vi "Cleanup.vi"(8 "error in (no error)":errorcluster, 11 "Vecto in":refnum<class "Vecto.lvclass">) -> (0 "error out":errorcluster)   [LabVIEW 2020, in "Vecto.lvlib" / "Vecto.lvclass"]
uses:
  Vecto.lvclass
  lv-http-server/HTTP Server/Server/Server.lvclass
  VectoService/VectoInfo.lvclass
  InfoService/NodeStatus.lvclass
  DiscoveryService/DiscoveryService.lvclass
  SequenceCountService/SequenceCountService.lvclass
  RemoteDataService/RemoteDataService.lvclass
  ChannelService/ChannelService.lvclass
  TCPMessaging/TCPMessaging.lvclass
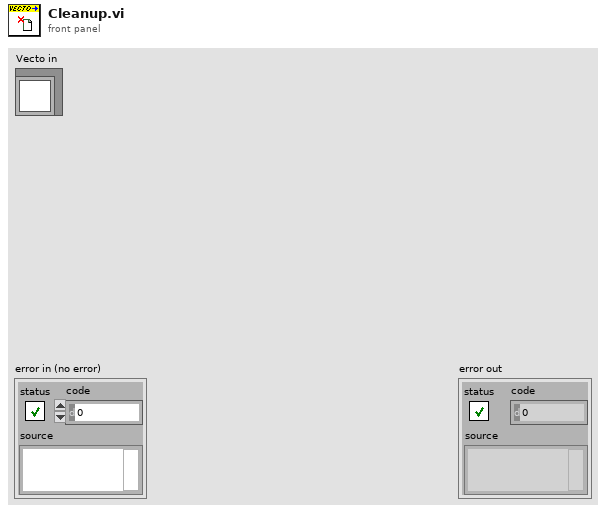
[diagram p1: front panel]
types:
  T1 = typedef "Vecto.lvlib/Vecto.lvclass/Local Services.ctl" = cluster{"InfoService":refnum<class "NodeStatus.lvclass">, "VectoService":refnum<class "VectoInfo.lvclass">, "ChannelService":refnum<class "ChannelService.lvclass">, "EventLogging":refnum<class "EventLoggingService.lvclass">}
  T2 = typedef "Vecto.lvlib/Vecto.lvclass/Remote Services.ctl" = cluster{"DiscoveryService":refnum<class "DiscoveryService.lvclass">, "SequenceCountService":refnum<class "SequenceCountService.lvclass">, "RemoteDataService":refnum<class "RemoteDataService.lvclass">, "TCPMessaging":refnum<class "TCPMessaging.lvclass">}
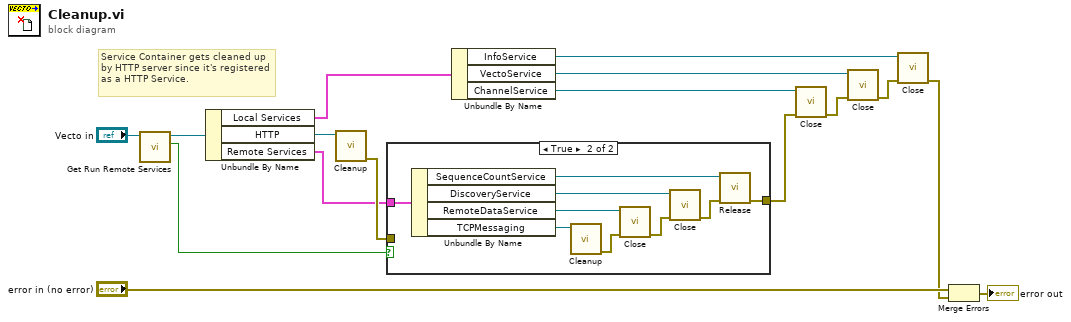
[diagram p0: block diagram]
diagram:
  # "Service Container gets cleaned up by HTTP server since it's registered as a HTTP Service."
  n1 = call "Get Run Remote Services.vi"("Vecto in"="Vecto in") -> ("Run Remote Services"=w7:bool, "Vecto out"=w8:refnum<class "Vecto.lvclass">)  [unwired: 8 in, 1 out]
  n2 = Unbundle By Name(w8) -> ("Local Services"=w14:T1, "HTTP"=w15:refnum<class "Server.lvclass">, "Remote Services"=w5:T2)
  n3 = call "Cleanup.vi"("Server in"=w15) -> ("error out"=w6:errorcluster)  [unwired: 10 in]
  n4 = case shown="True" w7 {
    tunnel: w6 -> [w17 _]
    tunnel: w5 -> [_ w26]
    tunnel: [w17 w22] -> w1
    frame False {
    }
    frame True {
      n5 = Unbundle By Name(w26) -> ("SequenceCountService"=w25:refnum<class "SequenceCountService.lvclass">, "DiscoveryService"=w24:refnum<class "DiscoveryService.lvclass">, "RemoteDataService"=w21:refnum<class "RemoteDataService.lvclass">, "TCPMessaging"=w19:refnum<class "TCPMessaging.lvclass">)
      n6 = call "Cleanup.vi"("TCPMessaging in"=w19) -> ("error out"=w18:errorcluster)  [unwired: 10 in]
      n7 = call "Close.vi"("error in (no error)"=w18, "RemoteDataService in"=w21) -> ("error out"=w20:errorcluster)  [unwired: 9 in]
      n8 = call "Close.vi"("error in (no error)"=w20, "DiscoveryService in"=w24) -> ("error out"=w23:errorcluster)  [unwired: 9 in]
      n9 = call "Release.vi"("error in (no error)"=w23, "SequenceCountService in"=w25) -> ("error out"=w22:errorcluster)  [unwired: 9 in]
    }
  }
  n10 = Unbundle By Name(w14) -> ("InfoService"=w12:refnum<class "NodeStatus.lvclass">, "VectoService"=w13:refnum<class "VectoInfo.lvclass">, "ChannelService"=w3:refnum<class "ChannelService.lvclass">)
  n11 = call "Close.vi"("error in (no error)"=w1, "ChannelService in"=w3) -> ("error out"=w2:errorcluster)  [unwired: 9 in]
  n12 = call "Close.vi"("error in (no error)"=w2, "VectoService in"=w13) -> ("error out"=w11:errorcluster)  [unwired: 9 in]
  n13 = call "Close.vi"("error in (no error)"=w11, "InfoService in"=w12) -> ("error out"=w4:errorcluster)  [unwired: 9 in]
  n14 = Merge Errors("error in (no error)", w4) -> (→"error out":errorcluster)
